vi "Auton Release Sequence.vi"(0 "PWM 5 Input":dbl, 2 "AI 5 Feedback":dbl, 3 "PWM 7 Input":dbl, 5 "AI 7 Feedback":dbl, 6 "Extension P":dbl=0.5, 7 "PWM 8 Input":dbl, 9 "PWM 9 Input":dbl, 10 "Enable Release Sequence":bool, 11 "DIO 3":bool) -> (14 "PWM 5 Output":dbl, 16 "PWM 7 Output":dbl, 18 "PWM 8 Output":dbl, 19 "PWM 9 Output":dbl)   [LabVIEW 2011]
uses:
  Robot Global Data.vi
panel:
  in  "PWM 5 Input 2":dbl
  in  "PWM 7 Input 2":dbl
  out "PWM 5 Output 2":dbl
  out "PWM 7 Output 2":dbl
  in  "PWM 8 Input 2":dbl
  out "PWM 8 Output 2":dbl
  in  "Release State 2":dbl
  in  "Enable Release Sequence 2":bool
  in  "AI 5 Feedback 2":dbl
  in  "AI 7 Feedback 2":dbl
  in  "DIO 4":bool
  out "Outer Release State 2":dbl
  in  "PWM 9 Input 2":dbl
  out "PWM 9 Output 2":dbl
  in  "Release Extension Power":dbl=0.2
  in  "Spit Out Speed":dbl=-0.4
  out "AI 5 Current":dbl
  out "AI 7 Current":dbl
  out "Outer Release State":dbl
  in  "Extension Release Extra":dbl=8.0
  in  "Release State":dbl
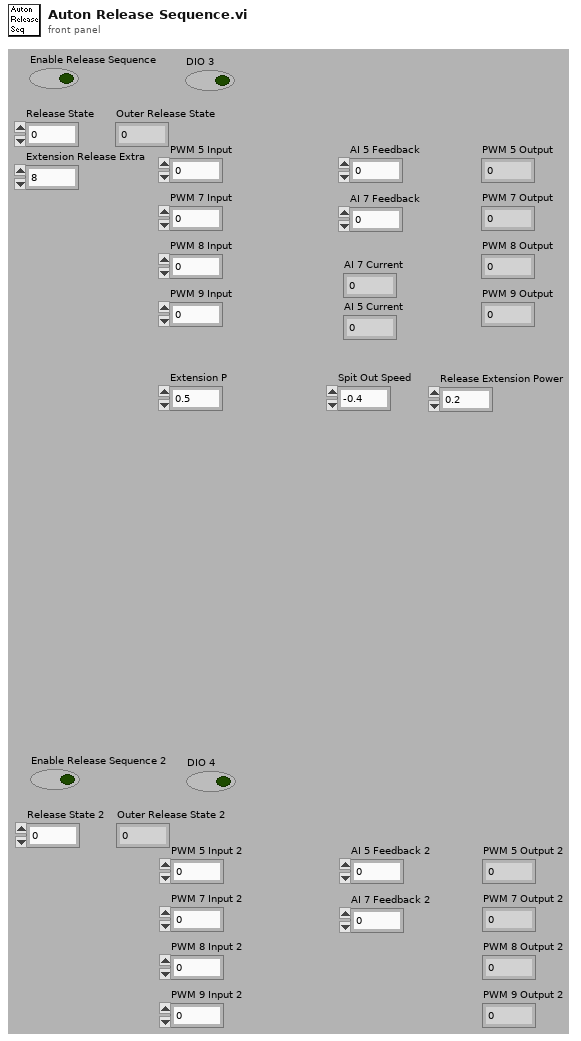
[diagram p1: front panel]
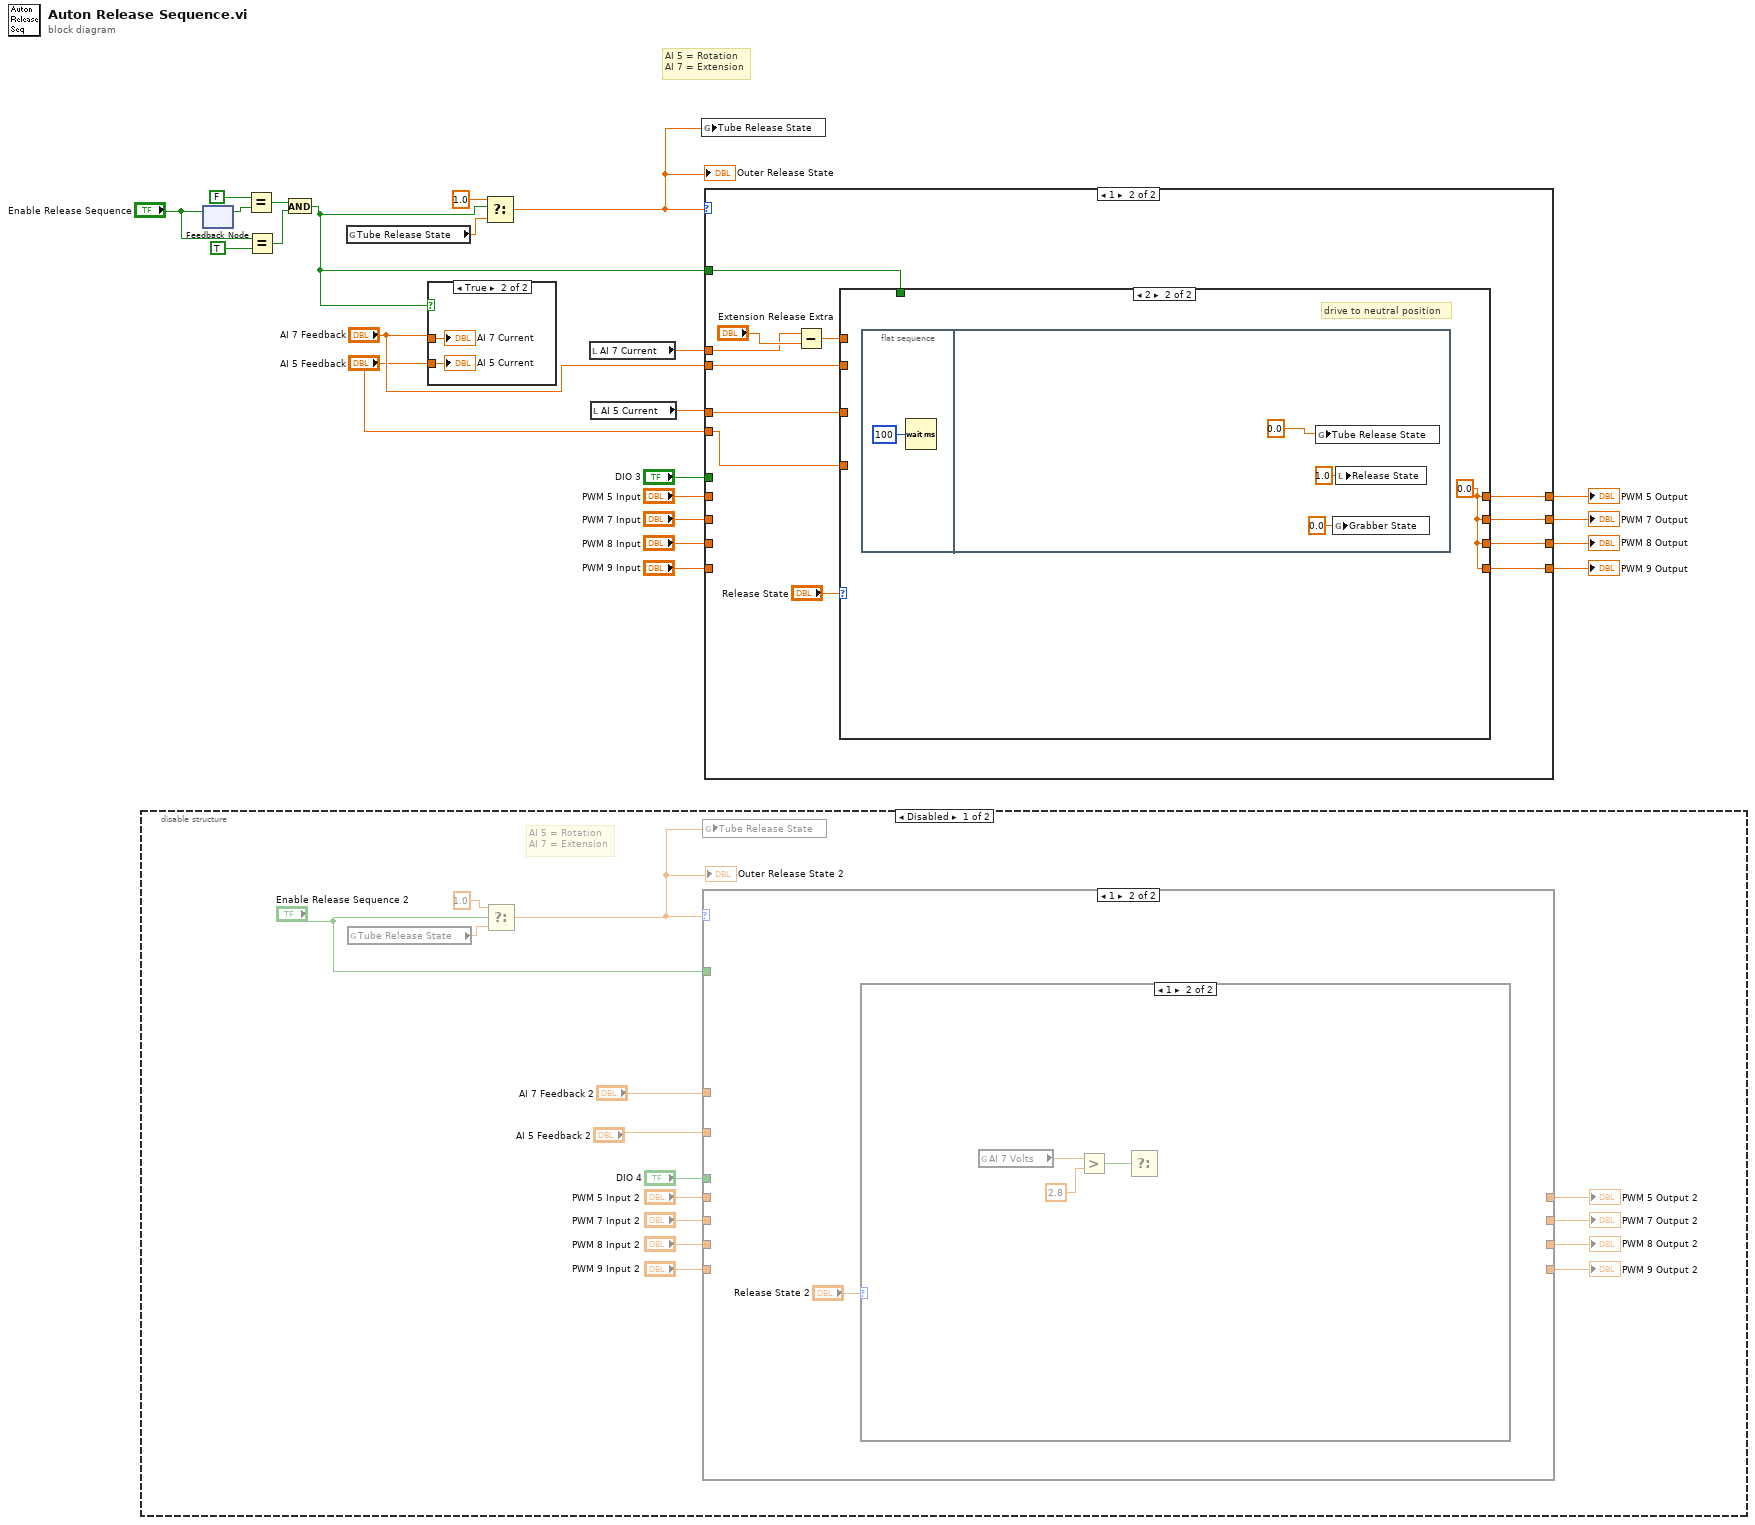
[diagram p0: block diagram]
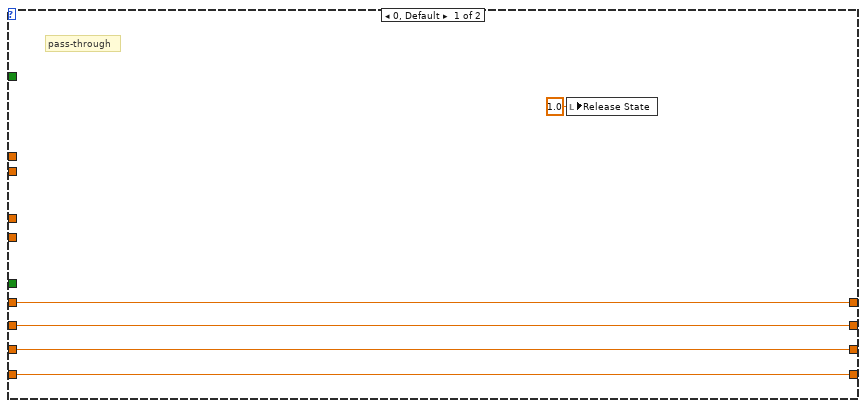
[diagram p3: hidden frame]
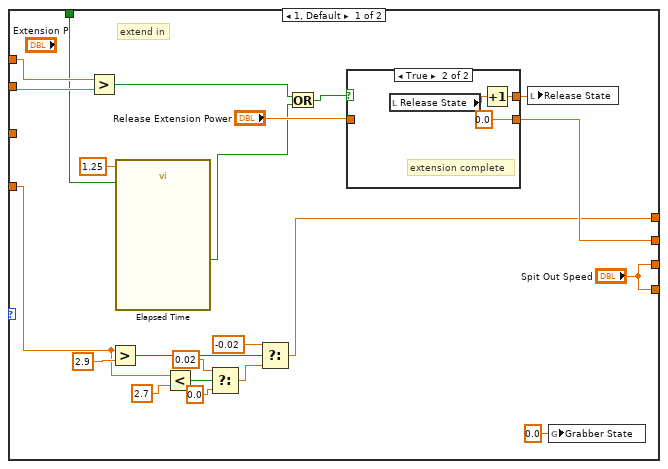
[diagram p4: hidden frame]
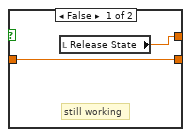
[diagram p5: hidden frame]
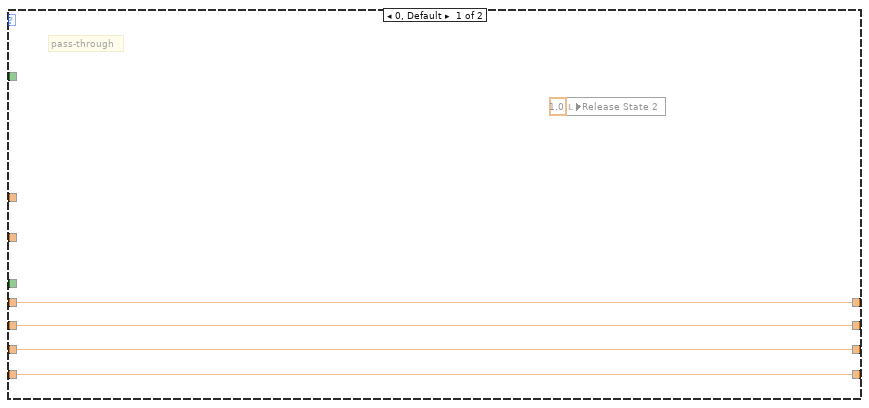
[diagram p6: hidden frame]
diagram:
  # "AI 5 = Rotation\nAI 7 = Extension"
  n1 = disable-structure shown="Disabled" {
    frame Disabled {
      # "AI 5 = Rotation\nAI 7 = Extension"
      n2 = global read "Robot Global Data.vi" "Tube Release State"() -> (w33:dbl)
      n3 = Select(t=1.0, s="Enable Release Sequence 2", f=w33) -> (s? t:f=w36:dbl)
      "Outer Release State 2" <- w36
      n4 = global write "Robot Global Data.vi" "Tube Release State"(w36) -> ()
      n5 = case shown="1" w36 {
        tunnel: [w43 _] -> w25
        tunnel: "PWM 5 Input 2" -> [w43 _]
        tunnel: "PWM 7 Input 2" -> [w42 _]
        tunnel: [w42 _] -> w28
        tunnel: "PWM 8 Input 2" -> [w41 _]
        tunnel: [w41 _] -> w30
        tunnel: "AI 7 Feedback 2" -> [_ _]
        tunnel: "AI 5 Feedback 2" -> [_ _]
        tunnel: "DIO 4" -> [_ _]
        tunnel: "PWM 9 Input 2" -> [w39 _]
        tunnel: [w39 _] -> w38
        tunnel: "Enable Release Sequence 2" -> [_ _]
        frame 0, Default {
          # "pass-through"
          n6 = local write "Release State 2"(1.0 ("Release State")) -> ()
        }
        frame 1 {
          n7 = case shown="1" "Release State 2" {
            frame 0, Default {
            }
            frame 1 {
              n8 = global read "Robot Global Data.vi" "AI 7 Volts"() -> (w47:dbl)
              n9 = Greater?(x=w47, y=2.8) -> (0:w45:bool)
              n10 = Select(s=w45) -> ()  [unwired: 2 in, 1 out]
            }
          }
        }
      }
      "PWM 5 Output 2" <- w25
      "PWM 7 Output 2" <- w28
      "PWM 8 Output 2" <- w30
      "PWM 9 Output 2" <- w38
    }
    frame Enabled {
    }
  }
  n11 = feedback-in #1("Enable Release Sequence") -> ()
  n12 = feedback #1() -> (w5:bool)  [unwired: 1 out]
  n13 = Equal?(x=FALSE, y=w5) -> (x = y?=w6:bool)
  n14 = Equal?(x="Enable Release Sequence", y=TRUE) -> (x = y?=w2:bool)
  n15 = And(x=w6, y=w2) -> (x .and. y?=w1:bool)
  n16 = global read "Robot Global Data.vi" "Tube Release State"() -> (w15:dbl)
  n17 = case shown="True" w1 {
    tunnel: "AI 7 Feedback" -> [_ w49]
    tunnel: "AI 5 Feedback" -> [_ w48]
    frame False {
    }
    frame True {
      "AI 7 Current" <- w49
      "AI 5 Current" <- w48
    }
  }
  n18 = Select(t=1.0, s=w1, f=w15) -> (s? t:f=w10:dbl)
  "Outer Release State" <- w10
  n19 = local read "AI 7 Current"() -> (w11:dbl)
  n20 = local read "AI 5 Current"() -> (w12:dbl)
  n21 = global write "Robot Global Data.vi" "Tube Release State"(w10) -> ()
  n22 = case shown="1" w10 {
    tunnel: [w54 w61] -> w23
    tunnel: "PWM 5 Input" -> [w54 _]
    tunnel: "PWM 7 Input" -> [w53 _]
    tunnel: [w53 w63] -> w20
    tunnel: "PWM 8 Input" -> [w52 _]
    tunnel: [w52 w59] -> w18
    tunnel: w11 -> [_ w56]
    tunnel: "AI 7 Feedback" -> [_ w64]
    tunnel: w12 -> [_ w62]
    tunnel: "AI 5 Feedback" -> [_ w60]
    tunnel: "DIO 3" -> [_ _]
    tunnel: "PWM 9 Input" -> [w50 _]
    tunnel: [w50 w58] -> w8
    tunnel: w1 -> [_ w55]
    frame 0, Default {
      # "pass-through"
      n23 = local write "Release State"(1.0 ("Release State")) -> ()
    }
    frame 1 {
      n24 = Subtract(x=w56, y="Extension Release Extra") -> (x-y=w65:dbl)
      n25 = case shown="2" "Release State" {
        tunnel: w65 -> [w85 _]
        tunnel: w64 -> [w84 _]
        tunnel: [w88 w94] -> w63
        tunnel: w62 -> [_ _]
        tunnel: [w77 w94] -> w61
        tunnel: w60 -> [w72 _]
        tunnel: ["Spit Out Speed" w94] -> w59
        tunnel: ["Spit Out Speed" w94] -> w58
        tunnel: w55 -> [w68 _]
        frame 1, Default {
          # "extend in"
          n26 = Greater?(x=w85, y=w84) -> (0:w80:bool)
          n27 = Greater?(x=w72, y=2.9) -> (0:w78:bool)
          n28 = call "Elapsed Time"("Time Target (s)"=1.25, "Reset"=w68) -> ("Time has Elapsed"=w75:bool)  [unwired: 3 in, 14 out]
          n29 = Less?(x=w72, y=2.7) -> (x < y?=w73:bool)
          n30 = Select(t=0.02, s=w73, f=0.0) -> (s? t:f=w74:dbl)
          n31 = Select(t=-0.02, s=w78, f=w74) -> (s? t:f=w77:dbl)
          n32 = Or(x=w80, y=w75) -> (x .or. y?=w81:bool)
          n33 = case shown="True" w81 {
            tunnel: [w90 0.0 ("Extension Point 5")] -> w88
            tunnel: "Release Extension Power" -> [w90 _]
            tunnel: [w89 w91] -> w87
            frame False {
              # "still working"
              n34 = local read "Release State"() -> (w89:dbl)
            }
            frame True {
              # "extension complete"
              n35 = local read "Release State"() -> (w92:dbl)
              n36 = Increment(x=w92) -> (x+1=w91:dbl)
            }
          }
          n37 = local write "Release State"(w87) -> ()
          n38 = global write "Robot Global Data.vi" "Grabber State"(0.0 ("Grabber State")) -> ()
        }
        frame 2 {
          w94 = 0.0 ("Extension Point 5")
          # "drive to neutral position"
          n39 = flat-sequence {
            frame #0 {
              n40 = Wait (ms)(milliseconds to wait=u32 100) -> ()  [unwired: 1 out]
            }
            frame #1 {
              n41 = global write "Robot Global Data.vi" "Tube Release State"(0.0 ("Enable Release Sequence")) -> ()
              n42 = global write "Robot Global Data.vi" "Grabber State"(0.0 ("Grabber State")) -> ()
              n43 = local write "Release State"(1.0 ("Release State")) -> ()
            }
          }
        }
      }
    }
  }
  "PWM 5 Output" <- w23
  "PWM 7 Output" <- w20
  "PWM 8 Output" <- w18
  "PWM 9 Output" <- w8
